vi "Create and Render Objects.vi"() -> ()   [LabVIEW 2023]
doc: "Demonstrates how to create objects based on basic geometries, change the drawing style, color the object and render it on the 3D Picture Control."
uses:
  <vilib>/Utility/miscctls.llb/LV3DPointTypeDef.ctl
  <vilib>/Analysis/baseanly.llb/Real Outer Product.vi
  <vilib>/Analysis/1siggen.llb/General Periodic Sinc.vi
  <vilib>/picture/3D Picture Control/Object/Create Object (drawable).vi
  <vilib>/picture/3D Picture Control/Object/Create Object (name).vi
  <vilib>/picture/3D Picture Control/Object/Add Object (no reference).vi
  <vilib>/picture/3D Picture Control/NI_3D Picture Control.lvlib
  <vilib>/Analysis/NI_AALBase.lvlib
panel:
  in  "Axis label?":bool=TRUE
  in  "Size":dbl=-1.0
  in  "show axis":bool=TRUE
  in  "Half plane?":bool=TRUE
  in  "Color":u32(colorbox)=16860
  in  "Draw Mode":T1(ring)=enum."Polygons"
  in  "Stop":bool
  in  "Geometries":T2(tab)
  in  "Box Length Y":sgl(slide)=1.0 scale=3.0..1e-06
  in  "Box Length X":sgl(slide)=1.0 scale=1e-06..3.0
  in  "Box Length Z":sgl(slide)=1.0 scale=1e-06..3.0
  in  "Sphere Radius":sgl(slide)=1.0 scale=0.1..3.0
  in  "Height":sgl(slide)=3.2222223 scale=1.0..5.0
  in  "Cone Radius":sgl(slide)=1.0 scale=1e-06..3.0
  in  "Cylinder Height":sgl(slide)=2.0 scale=0.1..5.0
  in  "Cylinder Radius":sgl(slide)=1.0 scale=0.1..2.0
  in  "Peak Height":dbl(slide)=2.0 scale=1.0..2.0
  in  "Row Interval":sgl=0.1 min=0.1 max=1 step=0.01
  in  "Column Interval":sgl=0.1 min=0.1 max=1 step=0.01
  in  "Base Height":sgl(slide)=1.0 scale=1.0..0.1
  in  "Pyramid Height":dbl(slide)=2.0 scale=0.0..5.0
  in  "Pyramid Base":dbl(slide)=1.0 scale=0.1..4.0
  in  "Pyramid Type":u16(ring)=1 items=["Triangular", "Square"]
  out "3D Picture":refnum<vi>(3d-picture)
  # "Overview: This VI demonstrates how to create and render objects in a 3D Picture.\nRequirements: LabVIEW Full Development System\nInstructions: \n1. Run the VI.\n2. Select the type of geometry (Box, Sphere, etc.) by selecting a tab on the Geometries tab control.\n3. Change the Draw Mode, Size, and Color to change the appearance of the object.\n4. Click Stop to stop the VI."
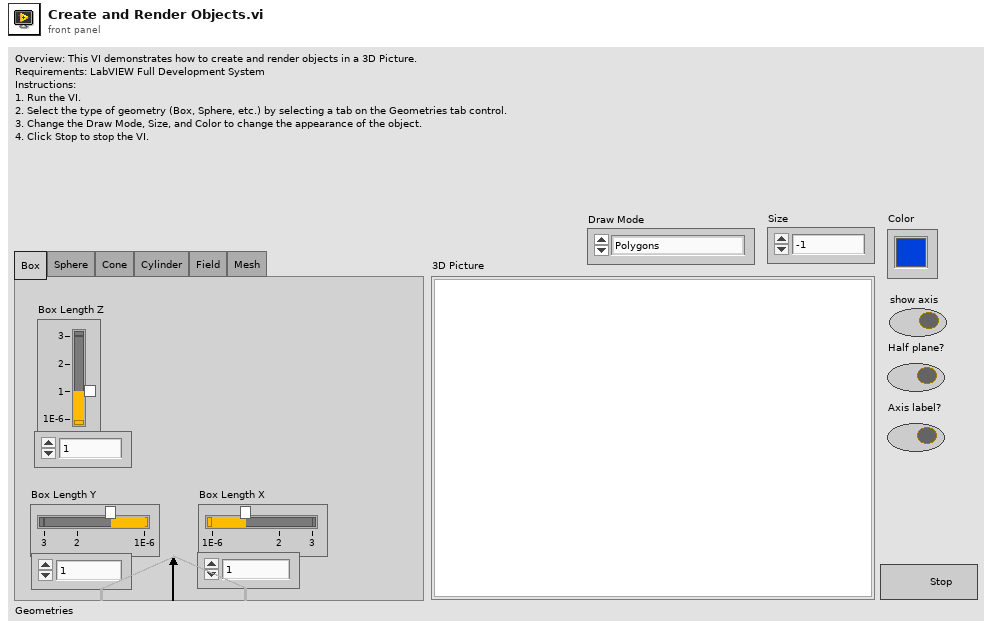
[diagram p1: front panel]
types:
  T1 = enum16{"Inherit Value", "Points", "Wireframe", "Polygons"}
  T2 = enum32{"Box", "Sphere", "Cone", "Cylinder", "Field", "Mesh"}
  T3 = typedef "LV3DPointTypeDef.ctl" = cluster{"X":sgl, "Y":sgl, "Z":sgl}
  T4 = enum16{"Overall", "Per Primitive", "Per Vertex", "Binding Off"}
  T5 = enum16{"Points", "Lines", "Line Strip", "Line Loop", "Triangles", "Triangle Strip", "Triangle Fan", "Quads", "Quad Strip", "Polygon"}
  T6 = typedef "NI_Matrix.lvlib/RealMatrix.ctl" = dbl[][]
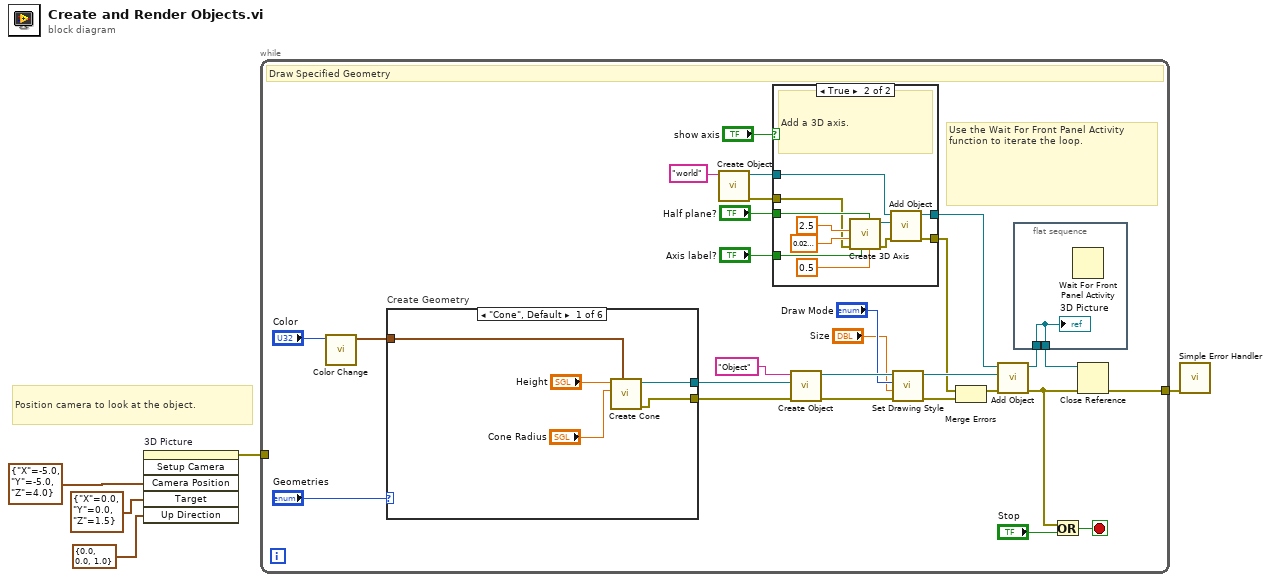
[diagram p0: block diagram]
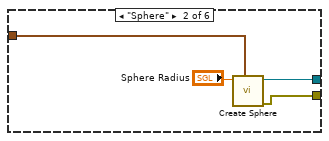
[diagram p3: hidden frame]
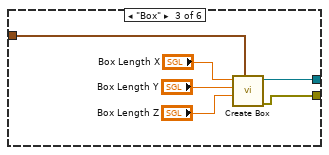
[diagram p4: hidden frame]
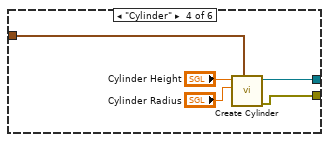
[diagram p5: hidden frame]
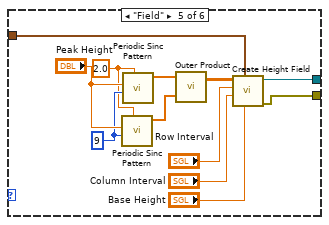
[diagram p6: hidden frame]
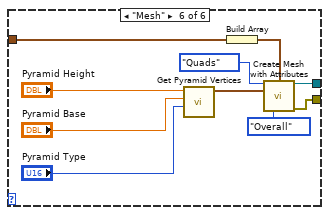
[diagram p7: hidden frame]
diagram:
  # "Position camera to look at the object."
  n1 = invoke on="3D Picture" class="SceneGraphDisp (strict)" method="Setup Camera"("Camera Position"=T3 {"X"=-5.0, "Y"=-5.0, "Z"=4.0}, "Target"=T3 {"X"=0.0, "Y"=0.0, "Z"=1.5} ("Camera Position"), "Up Direction"=T3 {"X"=0.0, "Y"=0.0, "Z"=1.0}) -> (error out=w5:errorcluster)  [unwired: 3 in, 5 out]
  n2 = while {
    tunnel: w5 -> [_]
    tunnel: [w8] -> w1
    stop <- w22 stop-if-true
    # "Use the Wait For Front Panel Activity function to iterate the loop."
    # "Draw Specified Geometry"
    n3 = call <vilib>:"Color Change.vi"("Color"="Color") -> ("RGBA"=w28:cluster{"R":sgl, "G":sgl, "B":sgl, "A":sgl})  [unwired: 10 in]
    n4 = case "Create Geometry" shown="\"Cone\", Default" "Geometries" {
      tunnel: [w51 w55 w61 w66 w78 w82] -> w30
      tunnel: w28 -> [w48 w53 w57 w63 w77 w85]
      tunnel: [w47 w52 w56 w62 w67 w80] -> w23
      frame "Cone", Default {
        n5 = call <vilib>:"Create Cone.vi"("Color"=w48, "Radius"="Cone Radius", "Height"="Height") -> ("error out"=w47:errorcluster, "New Cone Refnum"=w51:refnum<vi>)  [unwired: 7 in]
      }
      frame "Sphere" {
        n6 = call <vilib>:"Create Sphere.vi"("Color"=w53, "Radius"="Sphere Radius") -> ("error out"=w52:errorcluster, "New Sphere Refnum"=w55:refnum<vi>)  [unwired: 8 in]
      }
      frame "Box" {
        n7 = call <vilib>:"Create Box.vi"("Color"=w57, "Length Z"="Box Length Z", "Length Y"="Box Length Y", "Length X"="Box Length X") -> ("error out"=w56:errorcluster, "New Box Refnum"=w61:refnum<vi>)  [unwired: 6 in]
      }
      frame "Cylinder" {
        n8 = call <vilib>:"Create Cylinder.vi"("Color"=w63, "Radius"="Cylinder Radius", "Height"="Cylinder Height") -> ("error out"=w62:errorcluster, "New Cylinder Refnum"=w66:refnum<vi>)  [unwired: 7 in]
      }
      frame "Field" {
        w71 = 2.0 ("delay (s)")
        w72 = 9 ("order")
        n9 = call <vilib>:"Periodic Sinc Pattern.vi"("delay (s)"=w71, "order"=w72, "amplitude"="Peak Height") -> ("Periodic Sinc Pattern"=w74:dbl[])  [unwired: 7 in, 1 out]
        n10 = call <vilib>:"Periodic Sinc Pattern.vi"("delay (s)"=w71, "order"=w72, "amplitude"="Peak Height") -> ("Periodic Sinc Pattern"=w75:dbl[])  [unwired: 7 in, 1 out]
        n11 = call-poly <vilib>:"Outer Product.vi"("Y Vector"=w74, "X Vector"=w75) -> ("Outer Product"=w76:T6)  [unwired: 1 out]
        n12 = call <vilib>:"Create Height Field.vi"("Base Height"="Base Height", "Color"=w77, "Column Interval"="Column Interval", "Row Interval"="Row Interval", "Data"=w76) -> ("error out"=w67:errorcluster, "New Height Field Refnum"=w78:refnum<vi>)  [unwired: 5 in]
      }
      frame "Mesh" {
        n13 = call "Get Pyramid Vertices.vi"("Type"="Pyramid Type", "Base"="Pyramid Base", "Height"="Pyramid Height") -> ("Vertex Array"=w87:cluster{"X":dbl, "Y":dbl, "Z":dbl}[])  [unwired: 8 in]
        n14 = Build Array(w85) -> (w86:cluster{"R":sgl, "G":sgl, "B":sgl, "A":sgl}[])
        n15 = call <vilib>:"Create Mesh with Attributes.vi"("Draw Mode"=T5."Quads", "Color Array"=w86, "Vertex Array"=w87, "Normal Binding Mode"=T4."Overall") -> ("New Mesh Refnum"=w82:refnum<vi>, "error out"=w80:errorcluster)  [unwired: 10 in]
      }
    }
    n16 = call-poly <vilib>:"Create Object.vi"("Name"="world") -> ("error out"=w10:errorcluster, "Scene:New Object"=w11:refnum<vi>)  [unwired: 9 in]
    n17 = case shown="True" "show axis" {
      tunnel: [w35 w39] -> w26
      tunnel: "Half plane?" -> [_ w44]
      tunnel: [w34 w36] -> w15
      tunnel: "Axis label?" -> [_ w43]
      tunnel: w11 -> [w35 w41]
      tunnel: w10 -> [w34 w38]
      frame False {
        # "Pass an empty model when displaying no axis."
      }
      frame True {
        # "Add a 3D axis."
        n18 = call <vilib>:"Create 3D Axis.vi"("Character Size"=sgl 0.5, "Half plane?"=w44, "Axis label?"=w43, "error in (no error)"=w38, "Radius"=sgl 0.03, "Length"=sgl 2.5 ("Height")) -> ("error out"=w37:errorcluster, "New Object Refnum"=w40:refnum<vi>)  [unwired: 4 in]
        n19 = call-poly <vilib>:"Add Object.vi"("error in (no error)"=w37, "New Object In"=w40, "Scene Object In"=w41) -> ("error out"=w36:errorcluster, "Scene Object Out"=w39:refnum<vi>)  [unwired: 7 in]
      }
    }
    n20 = call-poly <vilib>:"Create Object.vi"("error in (no error)"=w23, "Geometry"=w30, "Name"="Object") -> ("error out"=w13:errorcluster, "Scene:New Object"=w21:refnum<vi>)  [unwired: 7 in]
    n21 = call <vilib>:"Set Drawing Style.vi"("error in (no error)"=w13, "Size"="Size", "Mode"="Draw Mode", "Scene Object In"=w21) -> ("error out"=w17:errorcluster, "Scene Object Out"=w20:refnum<vi>)  [unwired: 6 in]
    n22 = Merge Errors(w15, w17) -> (w16:errorcluster)
    n23 = call-poly <vilib>:"Add Object.vi"("error in (no error)"=w16, "New Object In"=w20, "Scene Object In"=w26) -> ("error out"=w9:errorcluster, "Scene Object Out"=w7:refnum<vi>)  [unwired: 7 in]
    n24 = flat-sequence {
      tunnel: w7 -> [w33]
      tunnel: [w33] -> w6
      frame #0 {
        n25 = Wait For Front Panel Activity() -> ()  [unwired: 3 in, 1 out]
        "3D Picture" <- w33
      }
    }
    n26 = Or(x=w9, y="Stop") -> (x .or. y?=w22:bool)
    n27 = Close Reference(reference=w6, error in (no error)=w9) -> (error out=w8:errorcluster)
  }
  n28 = call <vilib>:"Simple Error Handler.vi"("error in (no error)"=w1) -> ()  [unwired: 4 in, 5 out]
